vi "terminate_image_aquisition.vi"(0 "IMAQ Session In":refnum<k11>, 11 "error in (no error)":errorcluster) -> (15 "error out":errorcluster)   [LabVIEW 2023]
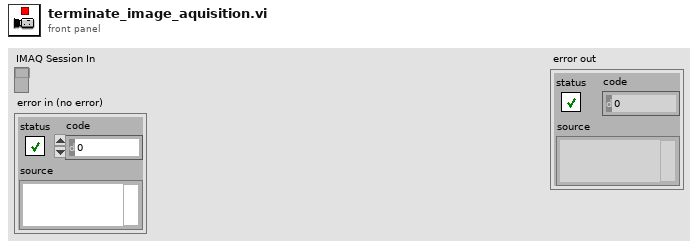
[diagram p1: front panel]
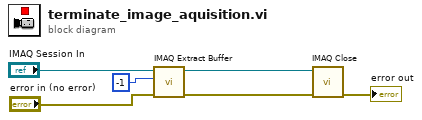
[diagram p0: block diagram]
diagram:
  n1 = call <vilib>:"IMAQ Extract Buffer.vi"("error in (no error)"="error in (no error)", "Buffer to extract"=-1, "IMAQ Session In"="IMAQ Session In") -> ("error out"=w5:errorcluster, "IMAQ Session Out"=w6:refnum<k11>)  [unwired: 3 in, 4 out]
  n2 = call <vilib>:"IMAQ Close.vi"("error in (no error)"=w5, "IMAQ Session In"=w6) -> ("error out"=→"error out":errorcluster)  [unwired: 9 in]
